vi "WriteData.vi"() -> ()   [LabVIEW 2015]
uses:
  <vilib>/addons/h5labview2/file/H5Fmode.ctl
  AcquisitionGlobals.vi
  NIDAQControls/StateGlobals.vi
  LiveImage_Global.vi
  <vilib>/addons/h5labview2/base/lib_path.vi
  <vilib>/addons/h5labview2/base/H5Equery.vi
  NIDAQControls/NIDAQGlobals.vi
  <vilib>/addons/h5labview2/attrib/H5Awrite.llb/H5Awrite.xnode
  <vilib>/addons/h5labview2/dataset/H5Dwrite.llb/H5Dwrite.xnode
  <vilib>/addons/h5labview2/base/hid_t.ctl
  <vilib>/addons/h5labview2/file/H5F.lvlib
  <vilib>/addons/h5labview2/dataset/H5D.lvlib
  <vilib>/addons/h5labview2/space/H5S.lvlib
panel:
  out "x-y":u32
  out "Frames Written":i32
  in  "error in (no error)":errorcluster
  out "error out":errorcluster
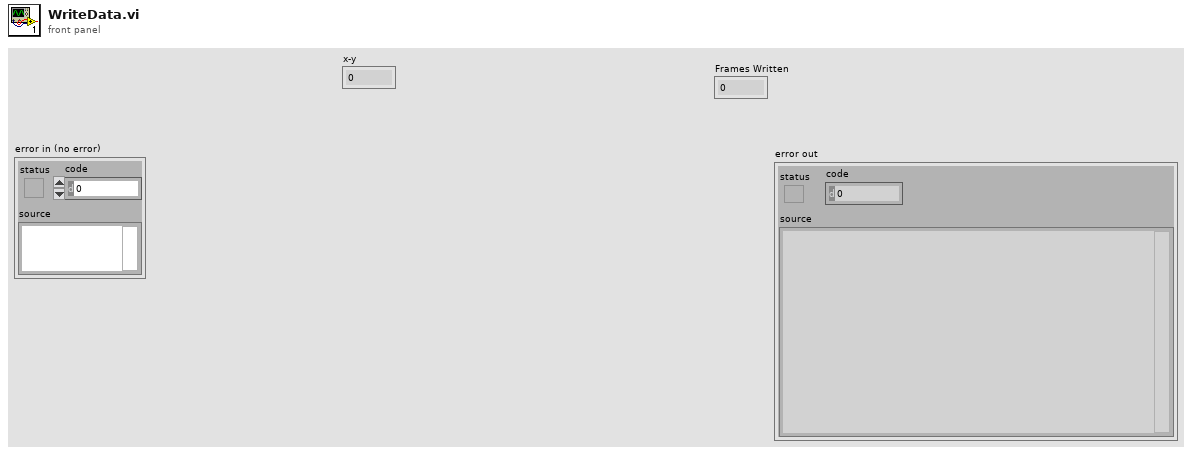
[diagram p1: front panel]
types:
  T1 = cluster{"Start or New Parameters?":bool, "Laser Mode":string, "Piezo Mode":string, "Begin Or End Acquisition":string, "Acquisition Time":dbl}
  T2 = typedef "H5F.lvlib/H5Fmode.ctl" = enum16{"read-only", "read-write", "overwrite", "create new", "open or create"}
  T3 = enum16{"Create", "Lossy Enqueue", "Enqueue", "Dequeue", "Destroy"}
  T4 = typedef "hid_t.ctl" = i32
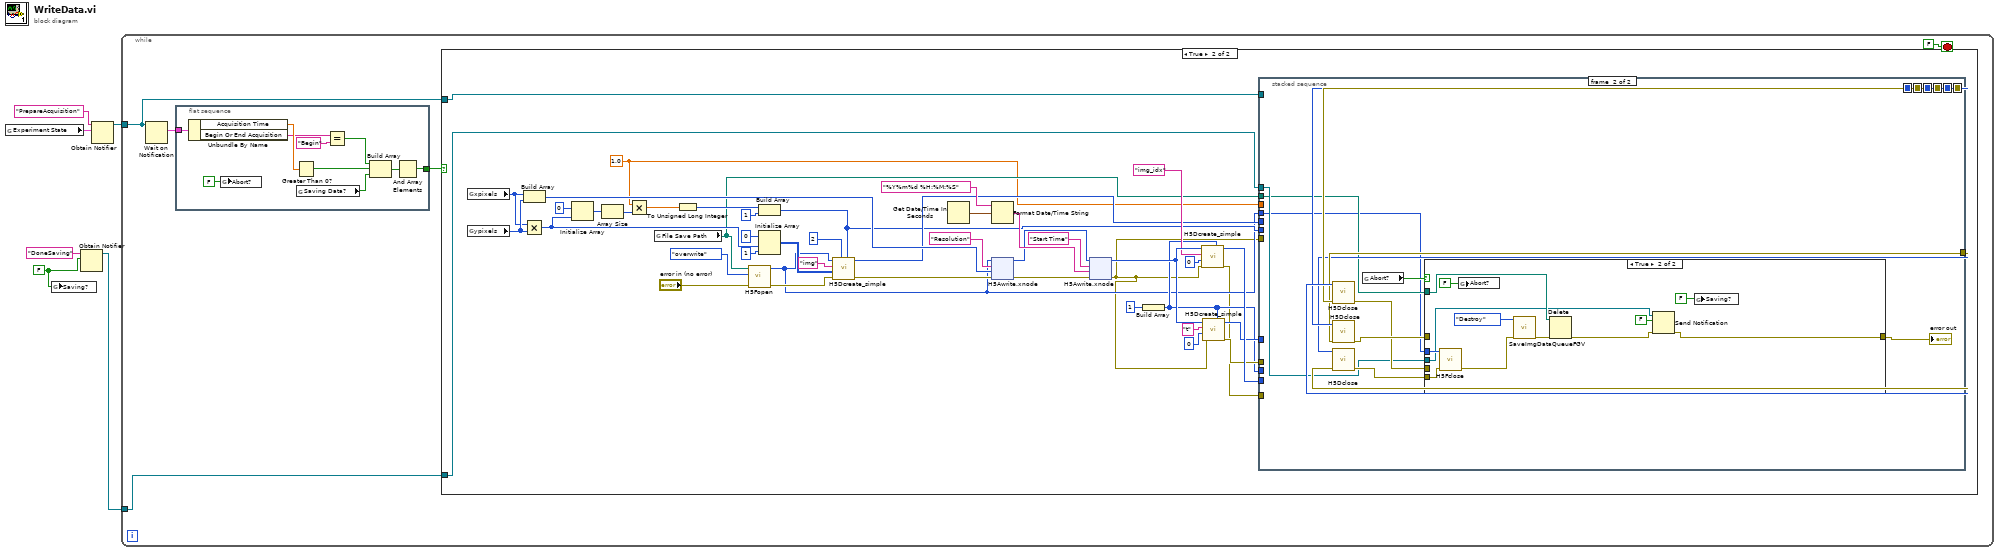
[diagram p0: block diagram]
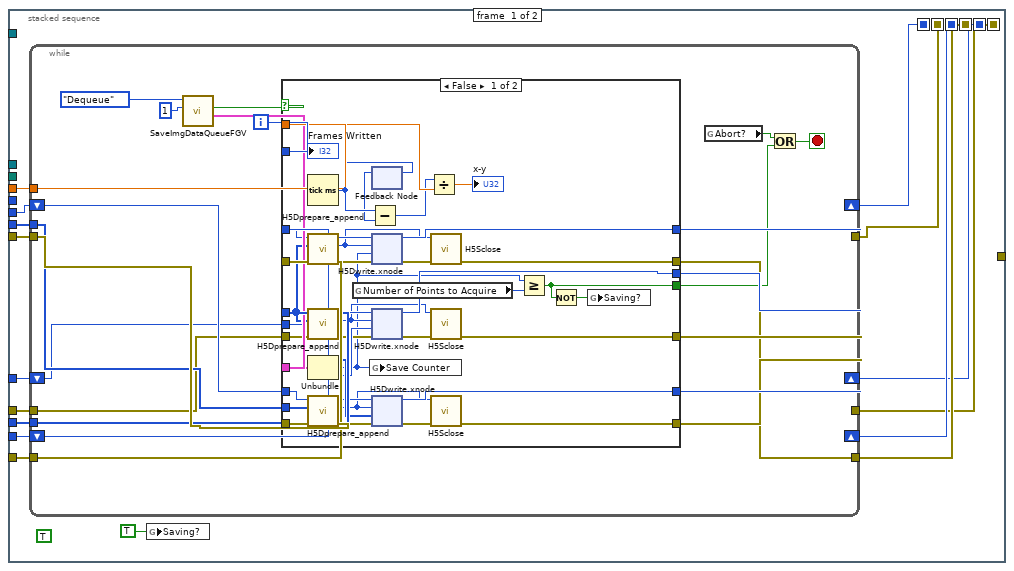
[diagram p3: hidden frame]
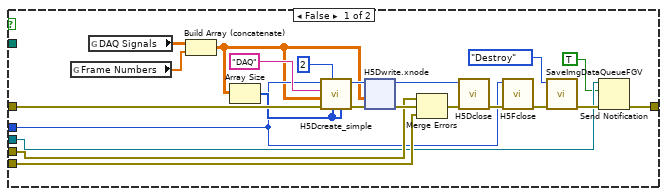
[diagram p5: hidden frame]
diagram:
  w2 = FALSE ("Saving?")
  n1 = global read "StateGlobals.vi" "Experiment State"() -> (w4:T1)
  n2 = global write "AcquisitionGlobals.vi" "Saving?"(w2) -> ()
  n3 = Obtain Notifier(name (unnamed)="DoneSaving", notification data type=w2) -> (notifier out=w1:refnum<notifier>)  [unwired: 2 in, 2 out]
  n4 = Obtain Notifier(name (unnamed)="PrepareAcquisition", notification data type=w4) -> (notifier out=w5:refnum<notifier>)  [unwired: 2 in, 2 out]
  n5 = while {
    tunnel: w5 -> [w9]
    tunnel: w1 -> [w7]
    stop <- FALSE stop-if-true
    n6 = Wait on Notification(notifier=w9) -> (notification=w11:T1)  [unwired: 3 in, 3 out]
    n7 = flat-sequence {
      tunnel: w11 -> [w21]
      tunnel: [w13] -> w8
      frame #0 {
        n8 = Unbundle By Name(w21) -> ("Acquisition Time"=w20:dbl, "Begin Or End Acquisition"=w18:string)
        n9 = global write "AcquisitionGlobals.vi" "Abort?"(FALSE ("Abort?")) -> ()
        n10 = Greater Than 0?(x=w20) -> (x > 0?=w16:bool)
        n11 = global read "AcquisitionGlobals.vi" "Saving Data?"() -> (w15:bool)
        n12 = Equal?(x=w18, y="Begin") -> (x = y?=w17:bool)
        n13 = Build Array(w17, w16, w15) -> (w14:bool[])
        n14 = And Array Elements(Boolean array=w14) -> (logical AND=w13:bool)
      }
    }
    n15 = case shown="True" w8 {
      tunnel: w9 -> [_ w66]
      tunnel: w7 -> [_ w65]
      frame False {
      }
      frame True {
        w22 = 1.0
        n16 = global read "LiveImage_Global.vi" "xpixels"() -> (w37:i32)
        n17 = global read "LiveImage_Global.vi" "ypixels"() -> (w38:i32)
        n18 = Multiply(x=w37, y=w38) -> (x*y=w42:i32)
        n19 = Build Array(w37, w38) -> (w39:i32[])
        n20 = Initialize Array(u16 0 ("element"), w42) -> (w35:u16[])
        n21 = Array Size(array=w35) -> (size(s)=w62:i32)
        n22 = Multiply(x=w22, y=w62) -> (x*y=w63:dbl)
        n23 = global read "AcquisitionGlobals.vi" "File Save Path"() -> (w26:path)
        n24 = To Unsigned Long Integer(number=w63) -> (unsigned 32bit integer=w64:u32)
        n25 = call <vilib>:"H5Fopen.vi"("error in (no error)"="error in (no error)", "mode (read-only)"=H5Fmode."overwrite", "path"=w26) -> ("error out"=w61:errorcluster, "ref out"=w25:T4)  [unwired: 7 in]
        n26 = Build Array(w64, 1 ("element")) -> (w27:u32[])
        n27 = Initialize Array(u16 0 ("element"), w42, 1 ("dimension size")) -> (w47:u16[][])
        n28 = call <vilib>:"H5Dcreate_simple.vi"("chunk size"=w27, "ndims"=2, "error in (no error)"=w61, "type in"=w47, "name"="img" ("Dataset Path"), "ref in"=w25) -> ("error out"=w50:errorcluster, "dset out"=w30:T4)  [unwired: 4 in]
        n29 = Get Date/Time In Seconds() -> (seconds since 1Jan1904=w57:timestamp)
        n30 = Format Date/Time String(time format string (%c)="%Y%m%d %H:%M:%S", seconds (now)=w57) -> (date/time string=w59:string)  [unwired: 1 in]
        n31 = xnode "H5Awrite.xnode"("error in (no error)"=w50, "data"=w39, "attrib name"="Resolution", "ref in"=w25) -> ("error out"=w55:errorcluster, "ref out"=w54:i32)  [unwired: 3 in, 1 out]
        n32 = xnode "H5Awrite.xnode"("error in (no error)"=w55, "data"=w59, "attrib name"="Start Time", "ref in"=w54) -> ("error out"=w24:errorcluster, "ref out"=w60:i32)  [unwired: 3 in, 1 out]
        n33 = Build Array(1) -> (w28:i32[])
        n34 = call <vilib>:"H5Dcreate_simple.vi"("chunk size"=w28, "error in (no error)"=w24, "type in"=0, "name"="img_idx" ("Dataset Path"), "ref in"=w60) -> ("error out"=w23:errorcluster, "dset out"=w32:T4)  [unwired: 5 in]
        n35 = call <vilib>:"H5Dcreate_simple.vi"("chunk size"=w28, "error in (no error)"=w24, "type in"=i64 0, "name"="t" ("Dataset Path"), "ref in"=w60) -> ("error out"=w29:errorcluster, "dset out"=w31:T4)  [unwired: 5 in]
        n36 = stacked-sequence {
          seq-local: [w103 _] -> [_ w248]
          seq-local: [w118 _] -> [_ w250]
          seq-local: [w117 _] -> [_ w249]
          seq-local: [w116 _] -> [_ w251]
          seq-local: [w115 _] -> [_ w247]
          seq-local: [w114 _] -> [_ w246]
          tunnel: w66 -> [_ _]
          tunnel: [_ w248] -> _
          tunnel: w65 -> [_ w245]
          tunnel: w32 -> [w112 _]
          tunnel: w31 -> [w111 _]
          tunnel: w30 -> [w110 _]
          tunnel: w24 -> [w109 _]
          tunnel: w29 -> [w108 _]
          tunnel: w28 -> [w107 _]
          tunnel: w27 -> [w106 _]
          tunnel: w26 -> [_ w242]
          tunnel: w25 -> [_ w241]
          tunnel: w23 -> [w105 _]
          tunnel: w22 -> [w104 _]
          frame #0 {
            (unwired) TRUE ("Unlimited  dataset (F)")
            n37 = while {
              tunnel: w109 -> [w139]
              shift-right: [w141] -> w117
              shift-left: w110 -> [w140]
              tunnel: [w128] -> w103
              shift-right: [w136] -> w116
              shift-left: w112 -> [w137]
              tunnel: [w127] -> w118
              tunnel: w105 -> [w138]
              tunnel: w107 -> [w132]
              tunnel: w106 -> [w135]
              shift-right: [w130] -> w115
              shift-left: w111 -> [w133]
              tunnel: w108 -> [w131]
              tunnel: [w129] -> w114
              tunnel: w104 -> [w126]
              i -> [w134]
              stop <- w119 stop-if-true
              n38 = call "SaveImgDataQueueFGV.vi"("timeout in ms (-1)"=1, "Action"=T3."Dequeue") -> ("Data Out"=w123:cluster{u16[], i32, i64}, "timed out?"=w122:bool)  [unwired: 7 in, 1 out]
              n39 = case shown="False" w122 {
                tunnel: [w180 w238] -> w141
                tunnel: w140 -> [w178 w238]
                tunnel: w139 -> [w176 w237]
                tunnel: w138 -> [w174 w239]
                tunnel: w137 -> [w173 w240]
                tunnel: [w170 w240] -> w136
                tunnel: w135 -> [w169 _]
                tunnel: w134 -> [w168 _]
                tunnel: w133 -> [w167 w236]
                tunnel: w132 -> [w166 _]
                tunnel: w131 -> [w165 w235]
                tunnel: [w161 w236] -> w130
                tunnel: [w159 w235] -> w129
                tunnel: [w156 w237] -> w128
                tunnel: [w152 w239] -> w127
                tunnel: [w151 _] -> w120
                tunnel: w126 -> [w148 _]
                tunnel: w123 -> [w145 _]
                frame False {
                  n40 = Tick Count (ms)() -> (millisecond timer value=w150:u32)
                  n41 = call <vilib>:"H5Dprepare_append.vi"("error in (no error)"=w174, "append dims"=w166, "dset in"=w173) -> ("error out"=w171:errorcluster, "space out"=w154:T4, "dset out"=w172:T4)  [unwired: 6 in]
                  n42 = call <vilib>:"H5Dprepare_append.vi"("error in (no error)"=w165, "append dims"=w166, "dset in"=w167) -> ("error out"=w162:errorcluster, "space out"=w158:T4, "dset out"=w163:T4)  [unwired: 6 in]
                  n43 = Unbundle(w145) -> (w179:u16[], w142:i32, w164:i64)
                  n44 = call <vilib>:"H5Dprepare_append.vi"("error in (no error)"=w176, "append dims"=w169, "dset in"=w178) -> ("error out"=w175:errorcluster, "space out"=w155:T4, "dset out"=w177:T4)  [unwired: 6 in]
                  n45 = global read "StateGlobals.vi" "Number of Points to Acquire"() -> (w143:i32)
                  n46 = global write "StateGlobals.vi" "Save Counter"(w142) -> ()
                  n47 = feedback #1() -> (w149:u32)  [unwired: 1 in]
                  n48 = Subtract(x=w150, y=w149) -> (x-y=w147:u32)
                  n49 = feedback-in #1(w150) -> ()
                  n50 = xnode "H5Dwrite.xnode"("error in (no error)"=w171, "data"=w142, "file space"=w154, "ref in"=w172) -> ("error out"=w153:errorcluster, "ref out"=w170:T4)  [unwired: 3 in, 1 out]
                  n51 = xnode "H5Dwrite.xnode"("error in (no error)"=w162, "data"=w164, "file space"=w158, "ref in"=w163) -> ("error out"=w160:errorcluster, "ref out"=w161:T4)  [unwired: 3 in, 1 out]
                  n52 = xnode "H5Dwrite.xnode"("error in (no error)"=w175, "data"=w179, "file space"=w155, "ref in"=w177) -> ("error out"=w157:errorcluster, "ref out"=w180:T4)  [unwired: 3 in, 1 out]
                  n53 = Divide(x=w147, y=w148) -> (x/y=→"x-y":dbl)
                  n54 = call <vilib>:"H5Sclose.vi"("error in (no error)"=w153, "space in"=w154) -> ("error out"=w152:errorcluster)  [unwired: 9 in]
                  n55 = call <vilib>:"H5Sclose.vi"("error in (no error)"=w160, "space in"=w158) -> ("error out"=w159:errorcluster)  [unwired: 9 in]
                  n56 = call <vilib>:"H5Sclose.vi"("error in (no error)"=w157, "space in"=w155) -> ("error out"=w156:errorcluster)  [unwired: 9 in]
                  n57 = Greater Or Equal?(x=w142, y=w143) -> (x >= y?=w151:bool)
                  n58 = Not(x=w151) -> (.not. x?=w144:bool)
                  n59 = global write "AcquisitionGlobals.vi" "Saving?"(w144) -> ()
                  "Frames Written" <- w168
                }
                frame True {
                }
              }
              n60 = global read "AcquisitionGlobals.vi" "Abort?"() -> (w121:bool)
              n61 = Or(x=w121, y=w120) -> (x .or. y?=w119:bool)
            }
            n62 = global write "AcquisitionGlobals.vi" "Saving?"(TRUE ("Saving?")) -> ()
          }
          frame #1 {
            n63 = call <vilib>:"H5Dclose.vi"("error in (no error)"=w250, "dset in"=w251) -> ("error out"=w252:errorcluster)  [unwired: 9 in]
            n64 = call <vilib>:"H5Dclose.vi"("error in (no error)"=w248, "dset in"=w249) -> ("error out"=w254:errorcluster)  [unwired: 9 in]
            n65 = call <vilib>:"H5Dclose.vi"("error in (no error)"=w246, "dset in"=w247) -> ("error out"=w253:errorcluster)  [unwired: 9 in]
            n66 = global read "AcquisitionGlobals.vi" "Abort?"() -> (w244:bool)
            n67 = case shown="True" w244 {
              tunnel: w254 -> [w274 _]
              tunnel: w253 -> [w273 w303]
              tunnel: w252 -> [w266 _]
              tunnel: w241 -> [w264 w304]
              tunnel: [w257 w297] -> w243
              tunnel: w245 -> [w256 w296]
              tunnel: w242 -> [_ w306]
              frame False {
                n68 = global read "NIDAQGlobals.vi" "Frame Numbers"() -> (w262:dbl[])
                n69 = global read "NIDAQGlobals.vi" "DAQ Signals"() -> (w263:dbl[][])
                n70 = Build Array (concatenate)(w263, w262) -> (w261:dbl[][])
                n71 = Array Size(array=w261) -> (size(s)=w268:i32[])
                n72 = call <vilib>:"H5Dcreate_simple.vi"("max size"=w268, "initial size"=w268, "ndims"=2, "error in (no error)"=w274, "type in"=w261, "name"="DAQ" ("Dataset Path"), "ref in"=w264) -> ("error out"=w275:errorcluster, "dset out"=w269:T4)  [unwired: 3 in]
                n73 = xnode "H5Dwrite.xnode"("error in (no error)"=w275, "data"=w261, "ref in"=w269) -> ("error out"=w276:errorcluster, "ref out"=w270:i32)  [unwired: 4 in, 1 out]
                n74 = Merge Errors(w266, w276, w273) -> (w271:errorcluster)
                n75 = call <vilib>:"H5Dclose.vi"("error in (no error)"=w271, "dset in"=w270) -> ("error out"=w272:errorcluster)  [unwired: 9 in]
                n76 = call <vilib>:"H5Fclose.vi"("error in (no error)"=w272, "ref"=w264) -> ("error out"=w260:errorcluster)  [unwired: 9 in]
                n77 = call "SaveImgDataQueueFGV.vi"("error out"=w260, "Action"=T3."Destroy") -> ("error out 2"=w258:errorcluster)  [unwired: 7 in, 2 out]
                n78 = Send Notification(notification=TRUE, notifier=w256, error in (no error)=w258) -> (error out=w257:errorcluster)  [unwired: 1 out]
              }
              frame True {
                n79 = call <vilib>:"H5Fclose.vi"("error in (no error)"=w303, "ref"=w304) -> ("error out"=w302:errorcluster)  [unwired: 9 in]
                n80 = global write "AcquisitionGlobals.vi" "Abort?"(FALSE ("Abort?")) -> ()
                n81 = call "SaveImgDataQueueFGV.vi"("error out"=w302, "Action"=T3."Destroy") -> ("error out 2"=w301:errorcluster)  [unwired: 7 in, 2 out]
                n82 = Delete(path (use dialog)=w306, error in=w301) -> (error out=w298:errorcluster)  [unwired: 3 in, 2 out]
                n83 = Send Notification(notification=FALSE, notifier=w296, error in (no error)=w298) -> (error out=w297:errorcluster)  [unwired: 1 out]
                n84 = global write "AcquisitionGlobals.vi" "Saving?"(FALSE ("Saving?")) -> ()
              }
            }
            "error out" <- w243
          }
        }
      }
    }
  }
